vi "Multiple spectra.vi"() -> (0 "error out":errorcluster)   [LabVIEW 2021, in "Ceyear.lvlib"]
uses:
  <instrlib>/Ceyear/Ceyear.lvlib
  <instrlib>/Ceyear/Public/Configure/Configure lbd (Start Stop).vi
  <vilib>/Utility/file.llb/Write To Spreadsheet File (string).vi
  <instrlib>/Keithley 24XX/Keithley 24XX.lvlib
panel:
  in  "reverce":bool
  out "appended array":string[][](array[string])
  in  "Array smsr":dbl[](array[numeric])
  in  "Array 2nd peak wl":dbl[](array[numeric])
  in  "Array 1st peak wl":dbl[](array[numeric])
  in  "Limit [V]":dbl=4.0 format="%#.4f"
  out "keithly2400 connection":bool
  out "VCSEL error":errorcluster
  in  "VCSEL Serial Configuration":T1={"Baud Rate"=9600, "Parity"=0, "Data Bits"=8, "Stop Bits"=10, "Flow Control"=0} {"Flow Control" items=["None", "XON/XOFF", "RTS/CTS", "XON/XOFF & RTS/CTS", "DTR/DSR", "XON/XOFF & DTR/DSR"]; "Stop Bits" items=["1.0"=10, "1.5"=15, "2.0"=20]; "Data Bits" items=["7"=7, "8"=8]; "Parity" items=["None", "Odd", "Even", "Mark", "Space"]; "Baud Rate" items=["300"=300, "600"=600, "1200"=1200, "2400"=2400, "4800"=4800, "9600"=9600, "19200"=19200]}
  in  "VCSEL VISA resource name":refnum<visa-resource-name>="GPIB0::26::INSTR"
  in  "Exit":bool
  in  "osa_time_array":dbl[](array[numeric])=[950.0, 1350.0, 4400.0, 7500.0, 65600.0]
  out "Estimated time, min":dbl
  out "scale":u16(ring)=1 items=["LIN", "LOG"]
  out "Graphs array":cluster{"ArrayX":dbl[], "ArrayY":dbl[]}[](array[cluster]) {"ArrayY" format="%.2f"; "ArrayX" format="%.2f"}
  in  "current graph":u16(ring) items=["1", "2", "3", "4", "5"]
  out "ArrayY":dbl[](array[numeric])
  out "ArrayX":dbl[](array[numeric])
  out "VISA out":refnum<visa-resource-name>
  in  "start array meas":bool
  out "Progress":u8(slide) scale=0.0..100.0
  in  "Delete [mA]":dbl=0.5 caption="delete [mA]" format="%#.6f"
  in  "Delete":bool
  in  "Append":bool
  in  "Change":bool
  in  "Add [mA]":dbl=0.5 caption="add [mA]" format="%#.6f"
  out "Current meas array":dbl[](array[numeric])
  out "Points LVI":i32=21 caption="Points"
  in  "Step [mA] LVI":dbl=0.2 caption="Step [mA]" format="%#.10f"
  in  "Start [mA] LVI":dbl=0.1 caption="Start [mA]" format="%#.6f"
  in  "Stop [mA] LVI":dbl=4.1 caption="Stop [mA]" format="%#.2f"
  in  "single":bool
  in  "dl resolution, nm":u16(ring)=2 items=["0.02", "0.05", "0.1", "0.2", "0.5", "1", "2"]
  in  "apply":bool
  in  "sampling point":i32=2001
  in  "average times":i32=1
  in  "trace Read/Measurement":u16(ring) items=["Trace A", "Trace B", "Trace C", "Trace D", "Trace E"]
  in  "sensivity":u16(ring) items=["NORMAL", "MID", "HIGH1", "HIGH2", "HIGH3"]
  in  "L max (nm)":dbl=900.0 format="%.2f"
  in  "L min (nm)":dbl=880.0 format="%.2f"
  in  "Selecting folder LIV":path=path "Select Folder" caption="Selecting folder"
  in  "save":bool
  in  "Filename peak wl":string="OS_peak_wl"
  in  "Filename smsr":string="OS_smsr"
  in  "Filename all spectra":string="OS_all_spectra"
  in  "save peak wl":bool=TRUE
  in  "save smsr":bool=TRUE
  in  "save all spectra data":bool=TRUE
  out "SMSR":cluster{"Current meas array":dbl[], dbl[]}(graph)
  out "peak wl":cluster{"Current meas array":dbl[], dbl[]}[](graph)
  out "All spectras":cluster{"ArrayX":dbl[], "ArrayY":dbl[]}[](graph)
  # "OSA trace parameters"
  # "optical input 600--1700 nm"
  # "101-50001 points"
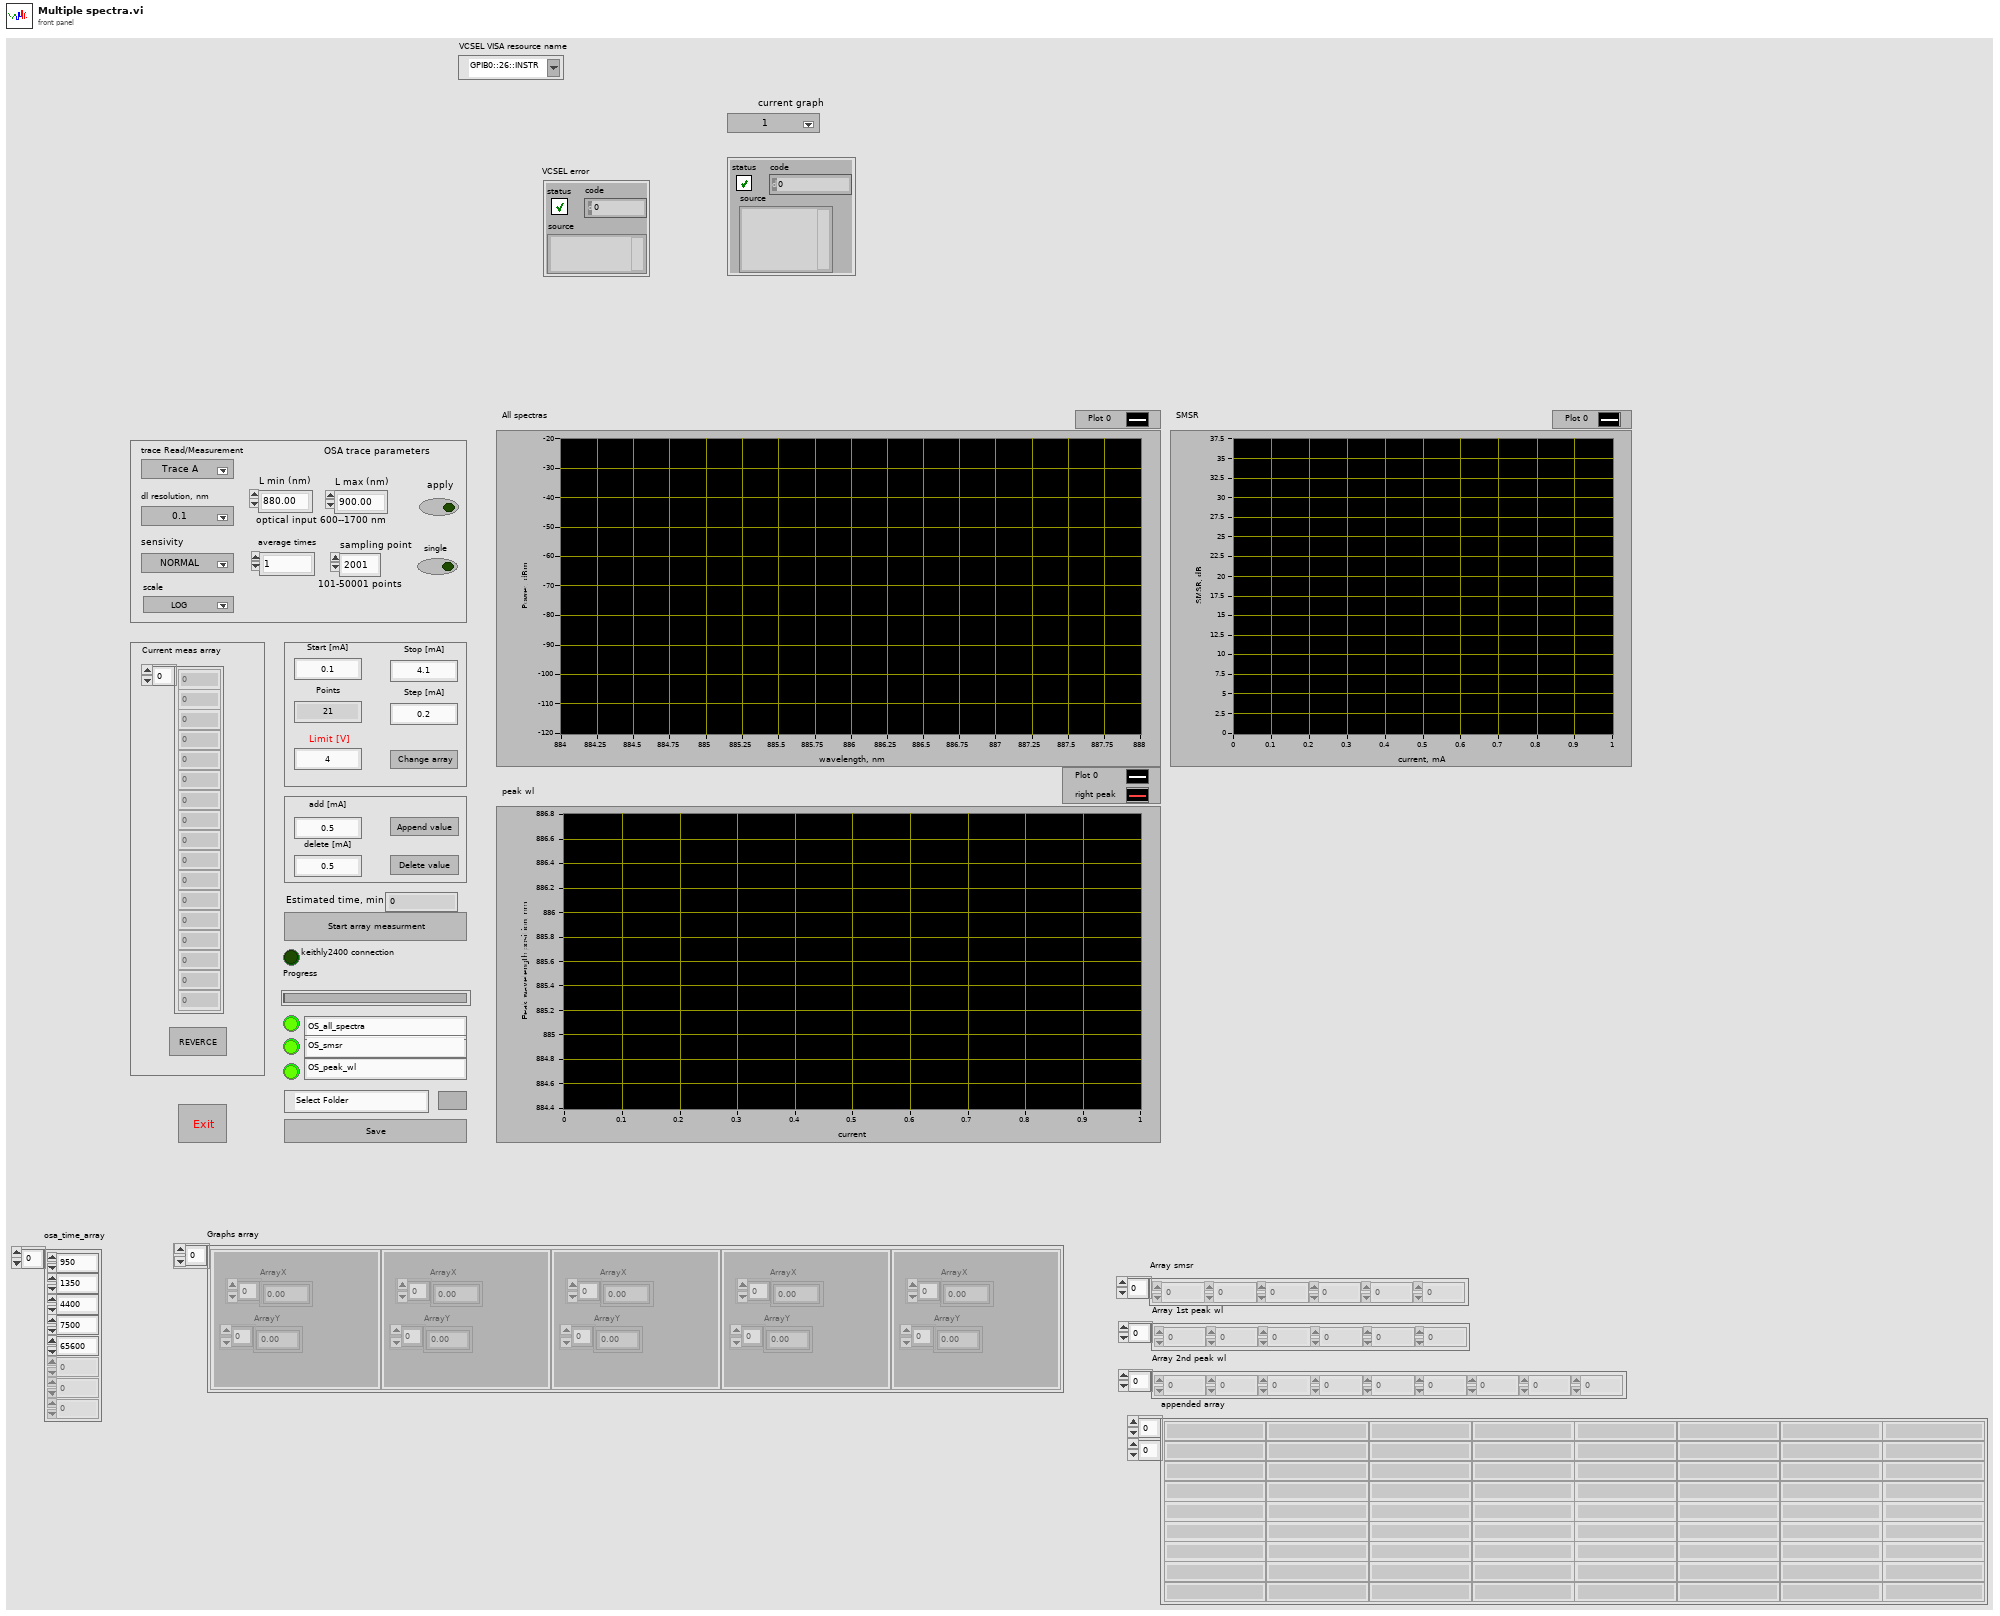
[diagram p1: front panel]
types:
  T1 = cluster{"Baud Rate":u32, "Parity":u16, "Data Bits":u16, "Stop Bits":u16, "Flow Control":u16}
  T2 = enum16{"Left Button", "Center Button", "Right Button", "Window Close"}
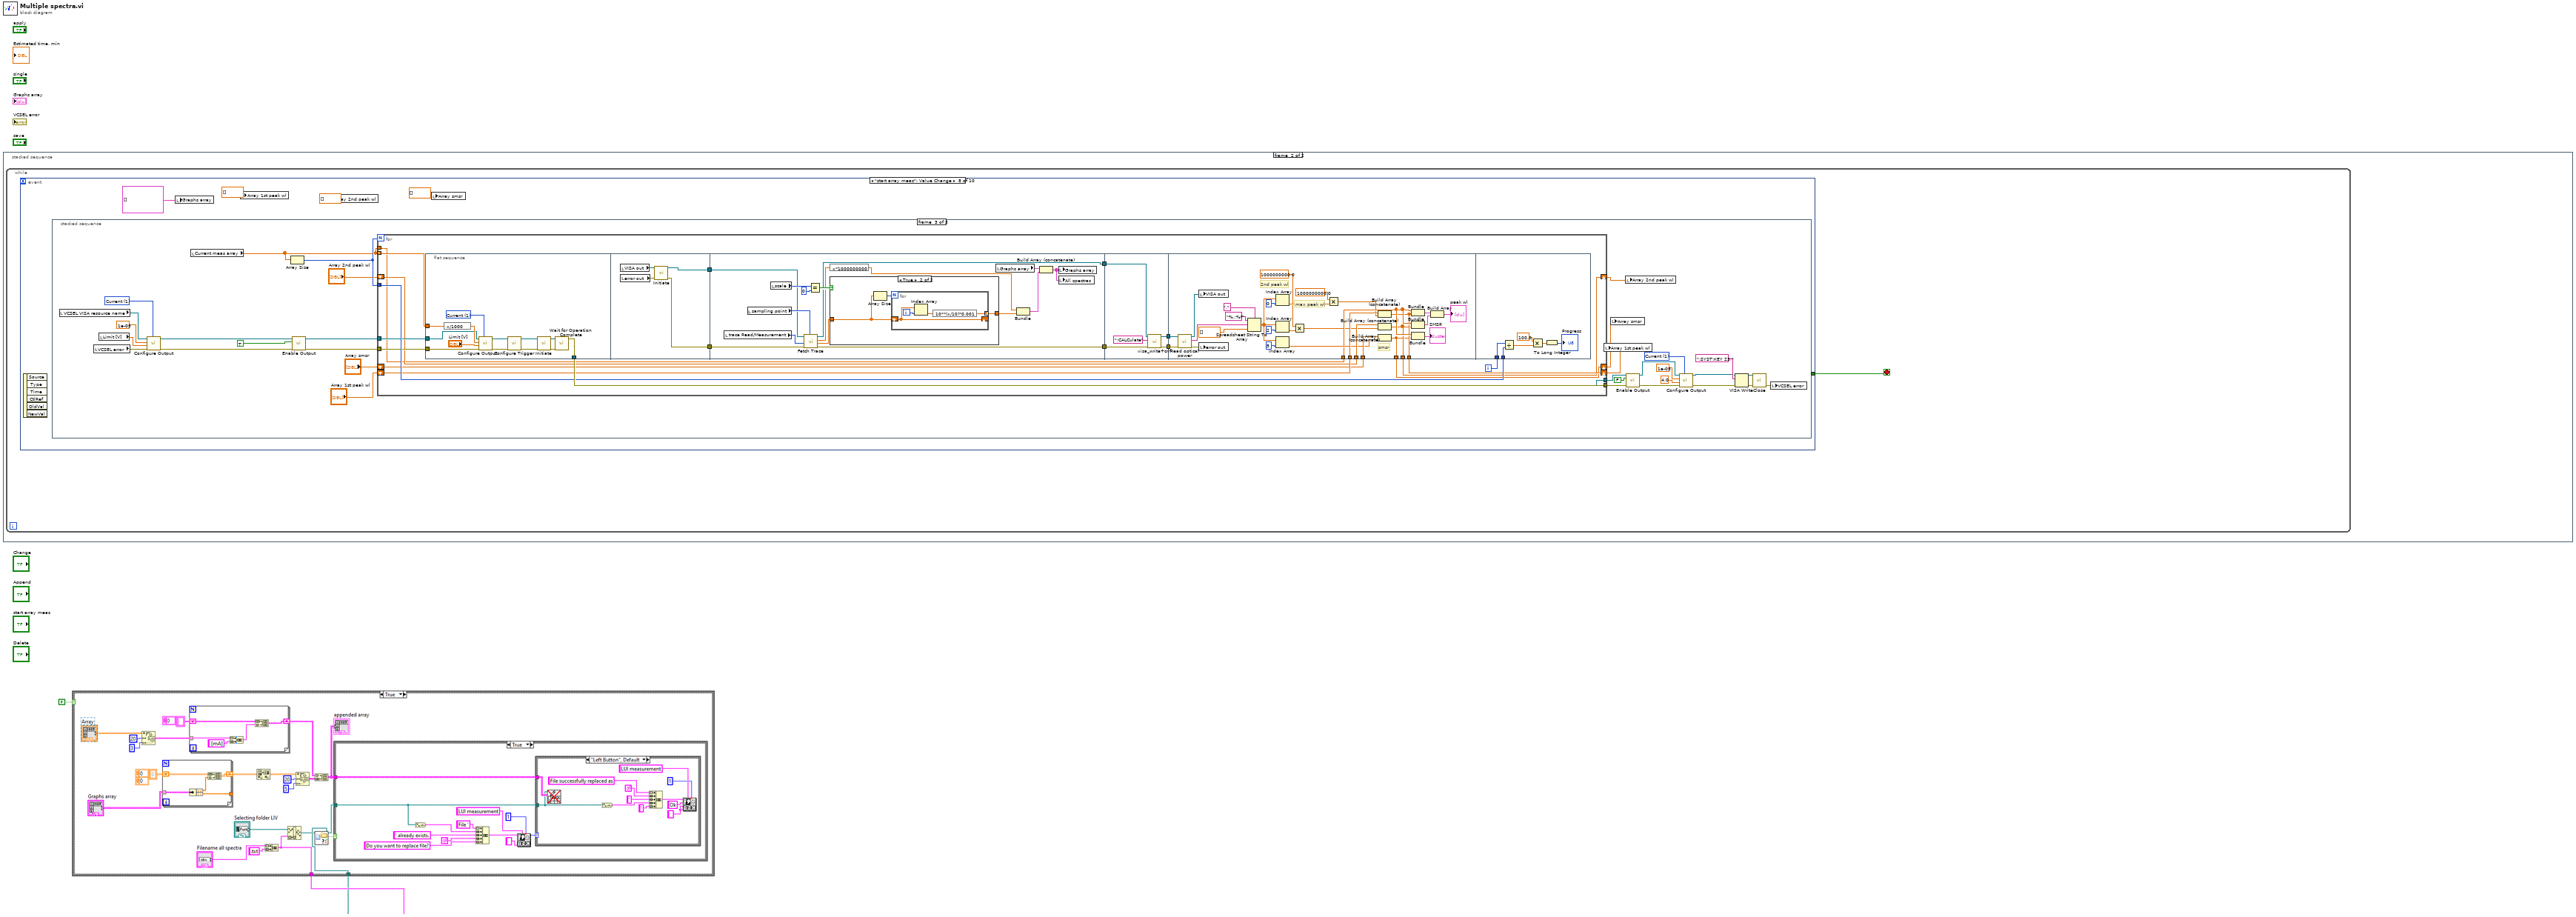
[diagram p0: block diagram]
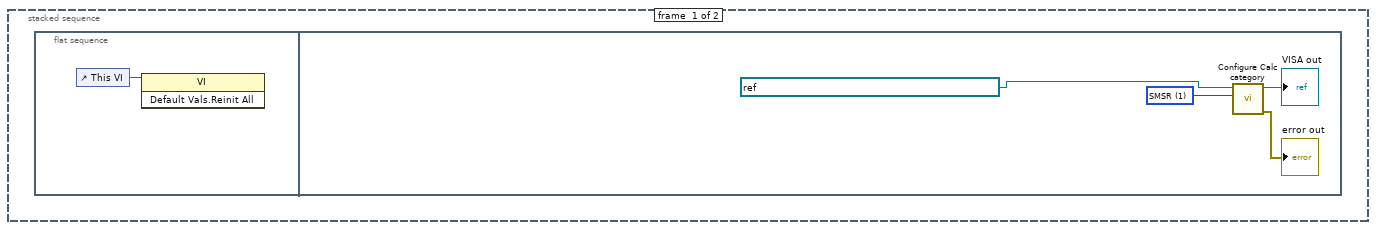
[diagram p2: hidden frame]
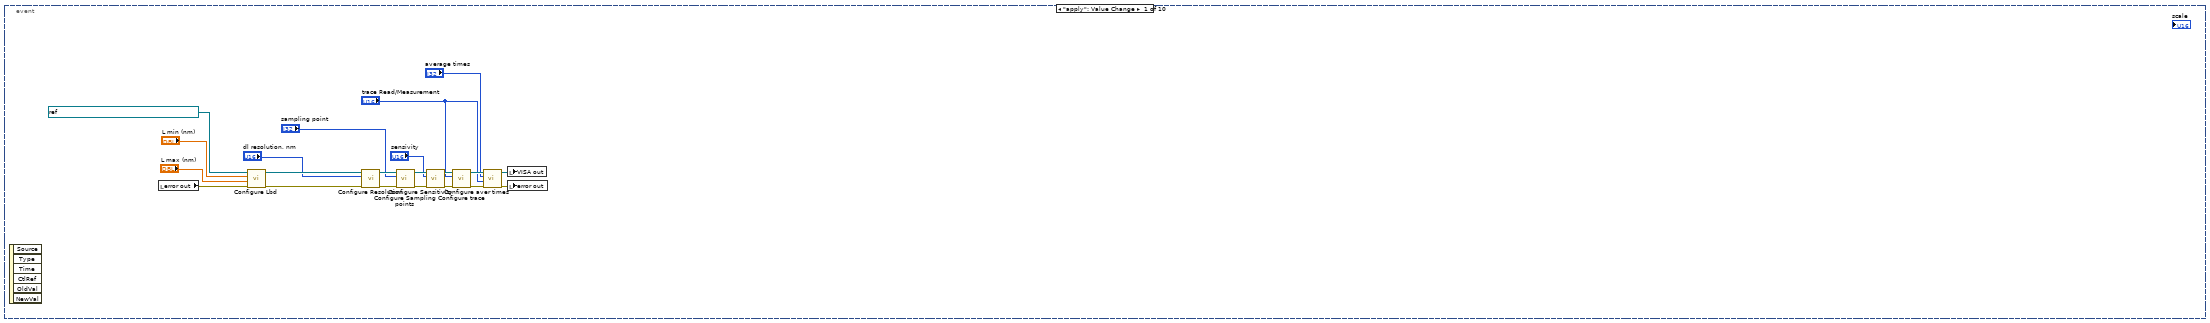
[diagram p3: hidden frame]
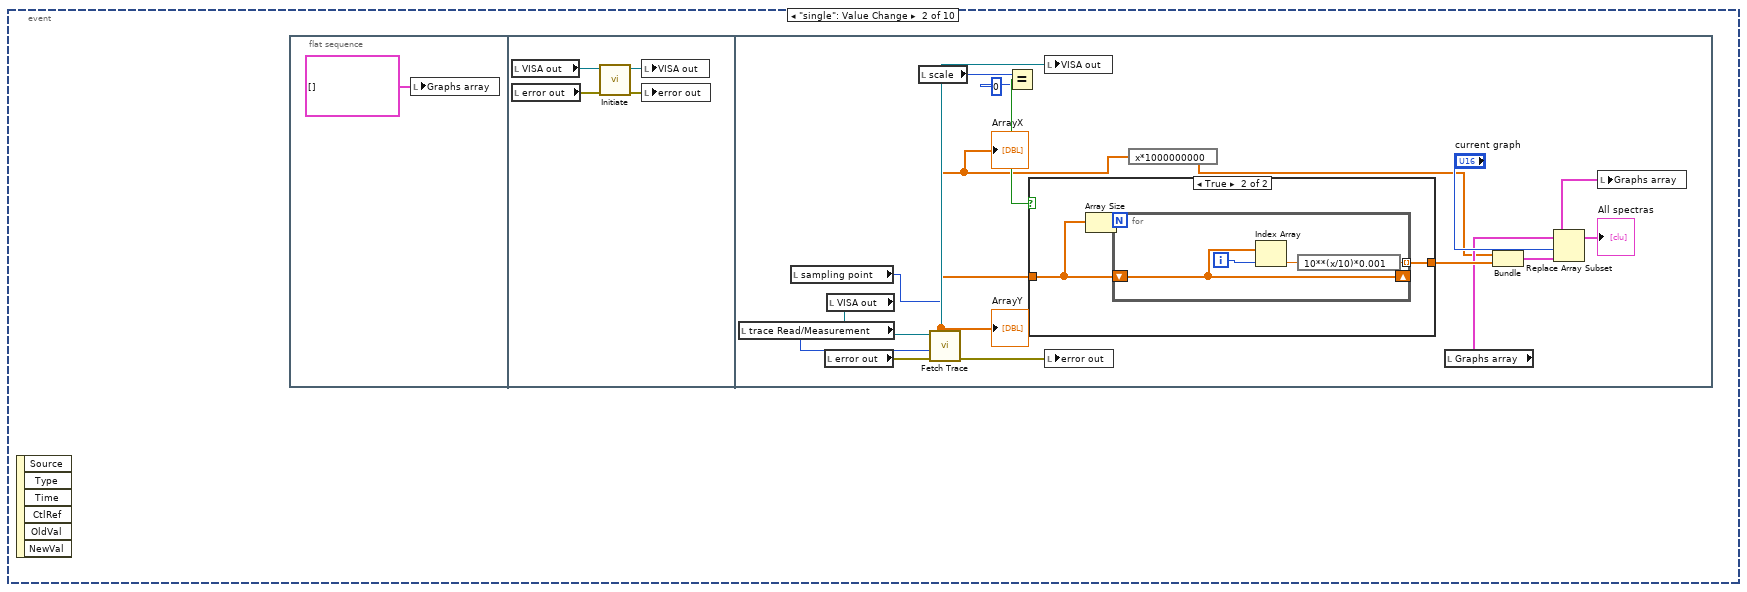
[diagram p4: hidden frame]
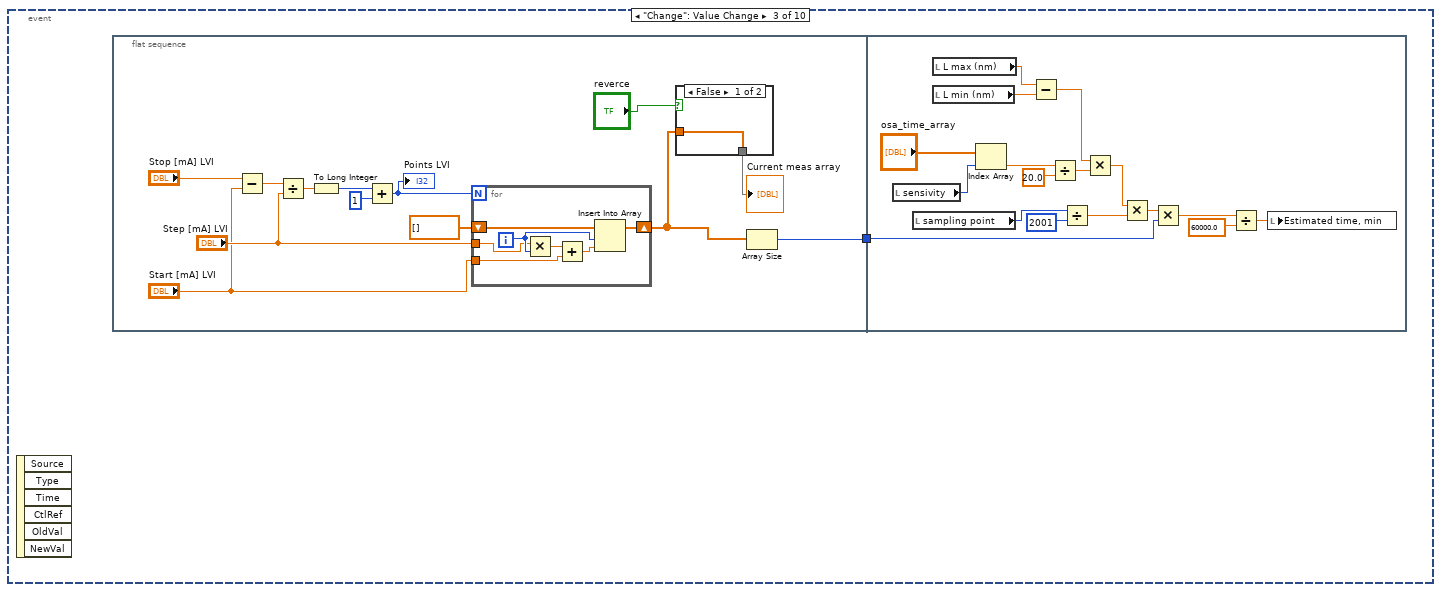
[diagram p6: hidden frame]
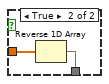
[diagram p7: hidden frame]
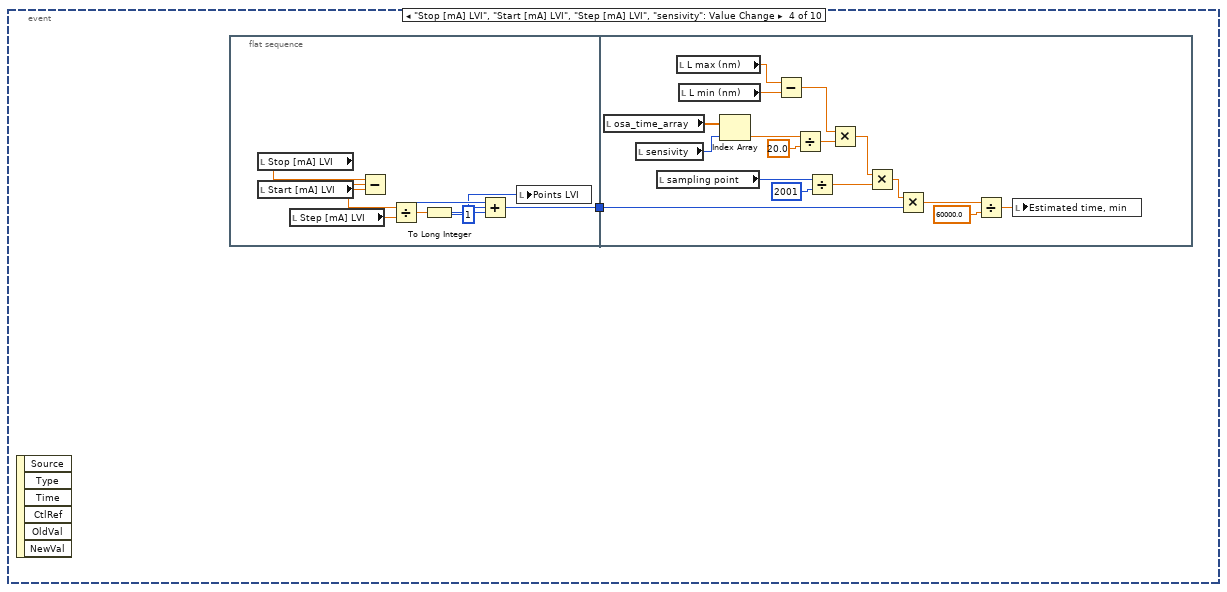
[diagram p8: hidden frame]
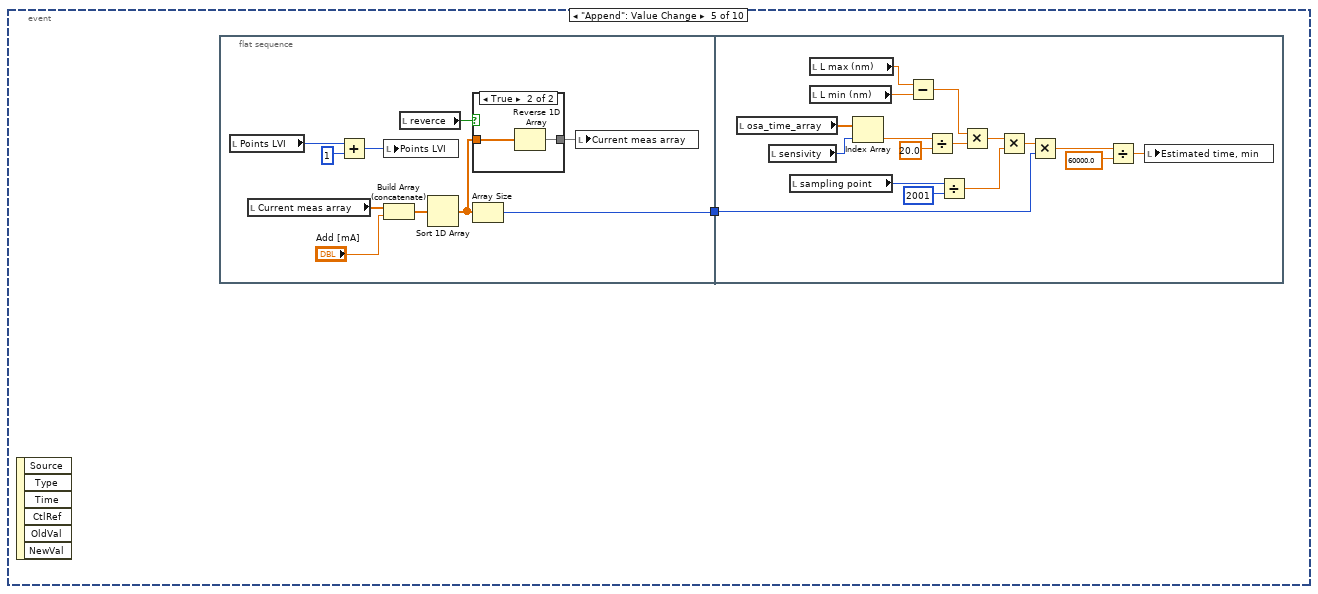
[diagram p9: hidden frame]
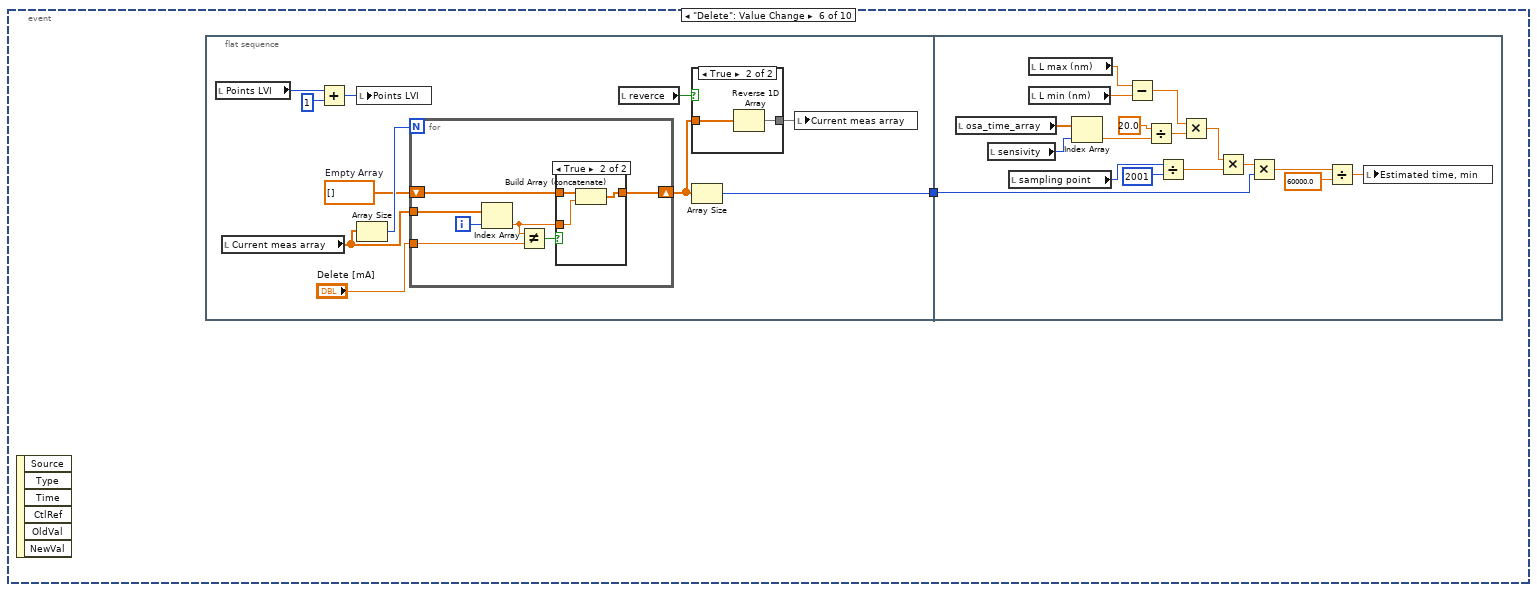
[diagram p11: hidden frame]
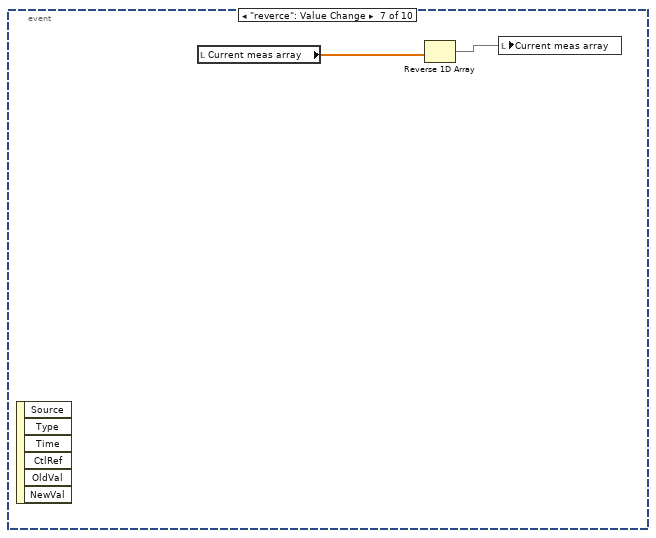
[diagram p14: hidden frame]
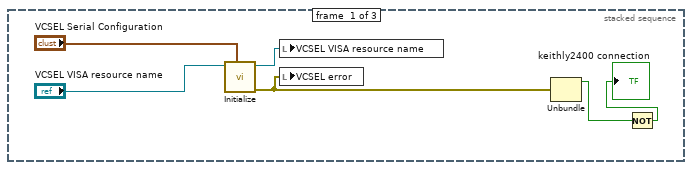
[diagram p15: hidden frame]
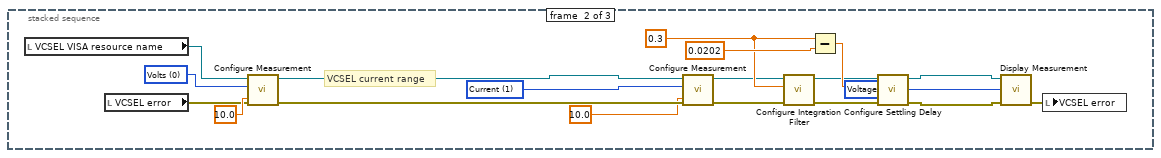
[diagram p16: hidden frame]
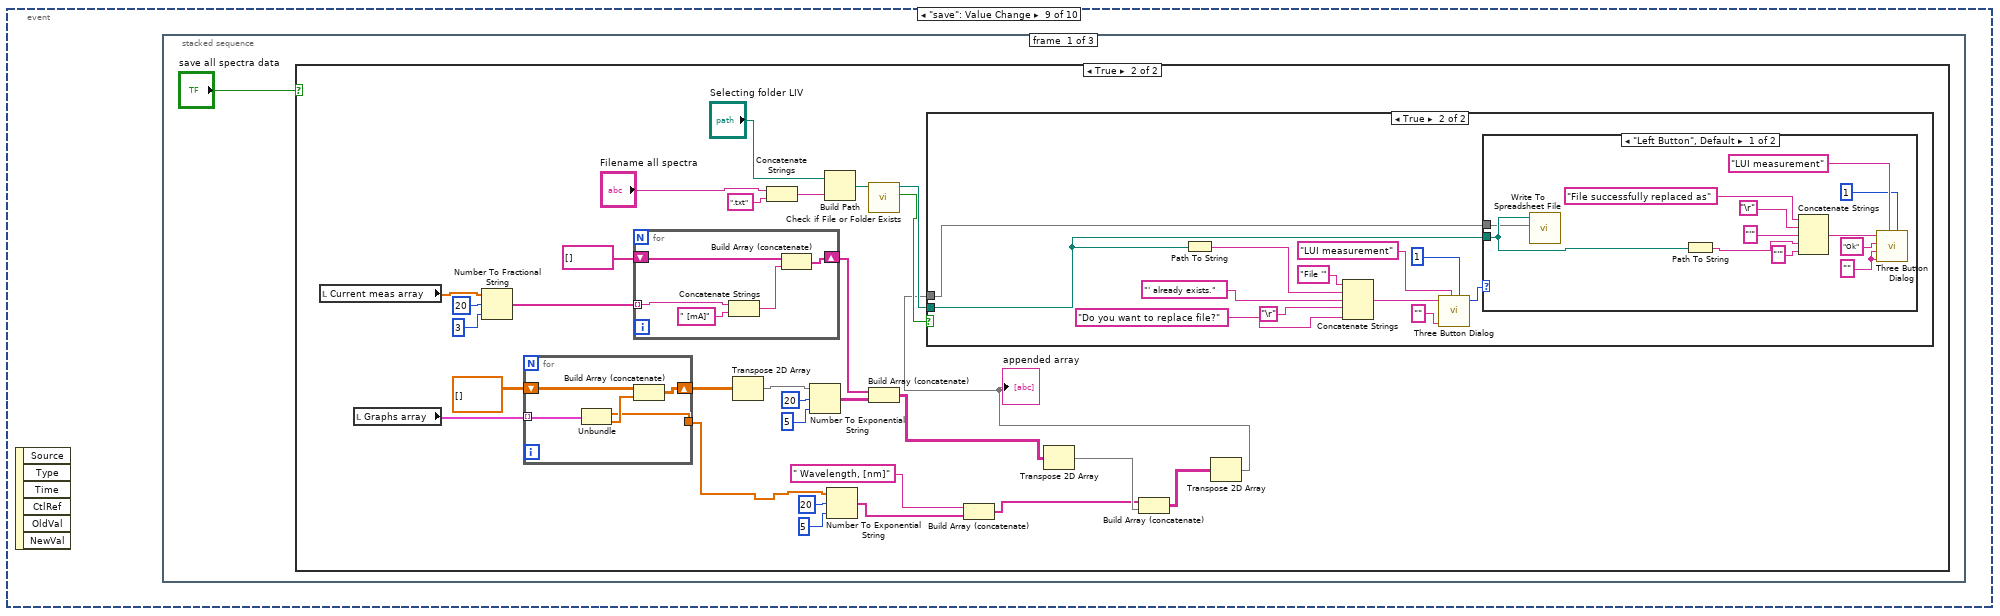
[diagram p18: hidden frame]
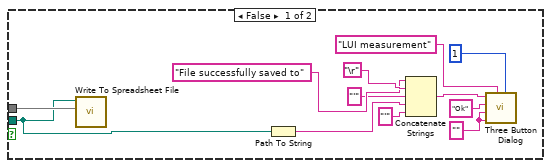
[diagram p20: hidden frame]
diagram:
  n1 = stacked-sequence {
    frame #0 {
      n2 = flat-sequence {
        frame #0 {
          n3 = control-ref of="This VI"() -> (w1:refnum<vi>)
          n4 = invoke class="VI" method="Default Vals.Reinit All"(reference=w1) -> ()  [unwired: 2 in, 3 out]
        }
        frame #1 {
          w5 = u16 1 items=["Power", "SMSR"] ("Category")
          n5 = call <instrlib>:"Configure Calc category.vi"("Category"=w5, "VISA resource name"=refnum<visa-resource-name> "TCPIP0::192.168.5.110::10001::SOCKET") -> ("error out"=→"error out":errorcluster, "VISA resource name out"=→"VISA out":refnum<visa-resource-name>)  [unwired: 7 in, 1 out]
        }
      }
    }
    frame #1 {
      n6 = while {
        stop <- w6 stop-if-true
        n7 = event shown="[7] \"start array meas\": Value Change" {
          selector: _ -> [_ _ _ _ _ _ _ _ _ _]
          dyn-events: _ -> [_ _ _ _ _ _ _ _ _ _]
          timeout: _ -> [_ _ _ _ _ _ _ _ _ _]
          tunnel: [_ _ _ _ _ _ _ _ _ w564] -> w6
          event "apply": Value Change {
            n8 = event-data() -> ()  [unwired: 1 in, 6 out]
            n9 = local read "error out"() -> (w15:errorcluster)
            n10 = call-poly <instrlib>:"Configure Lbd.vi"("error in (no error)"=w15, "Stop Frequency (nm)"="L max (nm)", "Start Frequency (nm)"="L min (nm)", "VISA resource name"=refnum<visa-resource-name> "TCPIP0::192.168.5.110::10001::SOCKET") -> ("error out"=w27:errorcluster, "VISA resource name out"=w22:refnum<visa-resource-name>)  [unwired: 6 in]
            n11 = call <instrlib>:"Configure Resolution.vi"("error in (no error)"=w27, "Resolution (nm)"="dl resolution, nm", "VISA resource name"=w22) -> ("error out"=w26:errorcluster, "VISA resource name out"=w23:refnum<visa-resource-name>)  [unwired: 7 in]
            n12 = call <instrlib>:"Configure Sampling points.vi"("error in (no error)"=w26, "Sampling points"="sampling point", "VISA resource name"=w23) -> ("error out"=w25:errorcluster, "VISA resource name out"=w24:refnum<visa-resource-name>)  [unwired: 7 in]
            n13 = call <instrlib>:"Configure Sensitivity.vi"("error in (no error)"=w25, "Sensse mode"="sensivity", "VISA resource name"=w24) -> ("error out"=w17:errorcluster, "VISA resource name out"=w16:refnum<visa-resource-name>)  [unwired: 7 in]
            n14 = call <instrlib>:"Configure trace.vi"("error in (no error)"=w17, "Trace"="trace Read/Measurement", "VISA resource name"=w16) -> ("error out"=w19:errorcluster, "VISA resource name out"=w18:refnum<visa-resource-name>)  [unwired: 7 in]
            n15 = call <instrlib>:"Configure aver times.vi"("error in (no error)"=w19, "Trace"="trace Read/Measurement", "Averaging times"="average times", "VISA resource name"=w18) -> ("error out"=w21:errorcluster, "VISA resource name out"=w20:refnum<visa-resource-name>)  [unwired: 6 in]
            n16 = local write "VISA out"(w20) -> ()
            n17 = local write "error out"(w21) -> ()
          }
          event "single": Value Change {
            n18 = event-data() -> ()  [unwired: 1 in, 6 out]
            n19 = flat-sequence {
              frame #0 {
                n20 = local write "Graphs array"(cluster{"ArrayX":dbl[], "ArrayY":dbl[]}[] [] ("Graphs array")) -> ()
              }
              frame #1 {
                n21 = local read "VISA out"() -> (w32:refnum<visa-resource-name>)
                n22 = local read "error out"() -> (w31:errorcluster)
                n23 = call <instrlib>:"Initiate.vi"("error in (no error)"=w31, "VISA resource name"=w32) -> ("error out"=w29:errorcluster, "VISA resource name out"=w30:refnum<visa-resource-name>)  [unwired: 8 in]
                n24 = local write "VISA out"(w30) -> ()
                n25 = local write "error out"(w29) -> ()
              }
              frame #2 {
                n26 = local read "trace Read/Measurement"() -> (w48:u16)
                n27 = local read "sampling point"() -> (w40:i32)
                n28 = local read "error out"() -> (w46:errorcluster)
                n29 = local read "VISA out"() -> (w47:refnum<visa-resource-name>)
                n30 = local read "scale"() -> (w42:u16)
                n31 = call <instrlib>:"Fetch Trace.vi"("Points"=w40, "error in (no error)"=w46, "Trace"=w48, "VISA resource name"=w47) -> ("error out"=w44:errorcluster, "Y array"=w43:dbl[], "X array"=w35:dbl[], "VISA resource name out"=w45:refnum<visa-resource-name>)  [unwired: 4 in]
                "ArrayX" <- w35
                "ArrayY" <- w43
                n32 = Equal?(x=w42, y=0) -> (x = y?=w41:bool)
                n33 = case shown="True" w41 {
                  tunnel: w43 -> [w50 w52]
                  tunnel: [w50 w51] -> w38
                  frame False {
                  }
                  frame True {
                    n34 = Array Size(array=w52) -> (size(s)=w53:i32)
                    n35 = for {
                      N: w53 -> [_]
                      shift-right: [w56] -> _
                      shift-left: w52 -> [w56]
                      tunnel: [w54] -> w51 mode=indexing
                      i -> [w57]
                      n36 = Index Array(array=w56, index=w57) -> (element=w55:dbl)
                      n37 = expression code="10**(x/10)*0.001"(w55) -> (w54:dbl)
                    }
                  }
                }
                n38 = local write "VISA out"(w45) -> ()
                n39 = local write "error out"(w44) -> ()
                n40 = expression code="x*1000000000"(w35) -> (w34:dbl[])
                n41 = local read "Graphs array"() -> (w37:cluster{"ArrayX":dbl[], "ArrayY":dbl[]}[])
                n42 = Bundle("X array"=w34, "Y array"=w38) -> (w36:cluster{"X array":dbl[], "Y array":dbl[]})  [unwired: 1 in]
                n43 = Replace Array Subset(array=w37, new element=w36, index="current graph") -> (w49:cluster{"ArrayX":dbl[], "ArrayY":dbl[]}[])
                "All spectras" <- w49
                n44 = local write "Graphs array"(w49) -> ()
              }
            }
          }
          event "Change": Value Change {
            n45 = event-data() -> ()  [unwired: 1 in, 6 out]
            n46 = flat-sequence {
              tunnel: [w67] -> w58
              tunnel: w58 -> [w98]
              frame #0 {
                n47 = Subtract(x="Stop [mA] LVI", y="Start [mA] LVI") -> (x-y=w70:dbl)
                n48 = Divide(x=w70, y="Step [mA] LVI") -> (x/y=w68:dbl)
                n49 = To Long Integer(number=w68) -> (32bit integer=w63:i32)
                n50 = Add(x=w63, y=1) -> (x+y=w64:i32)
                "Points LVI" <- w64
                n51 = for {
                  N: w64 -> [_]
                  shift-right: [w78] -> w61
                  shift-left: dbl[] [] ("Current meas array") -> [w81]
                  tunnel: "Step [mA] LVI" -> [w79]
                  tunnel: "Start [mA] LVI" -> [w76]
                  i -> [w80]
                  n52 = Multiply(x=w79, y=w80) -> (x*y=w77:dbl)
                  n53 = Add(x=w77, y=w76) -> (x+y=w75:dbl)
                  n54 = Insert Into Array(array=w81, index=w80, new element=w75) -> (w78:dbl[])
                }
                n55 = case shown="False" "reverce" {
                  tunnel: w61 -> [w72 w74]
                  tunnel: [w72 w73] -> w60
                  frame False {
                  }
                  frame True {
                    n56 = Reverse 1D Array(array=w74) -> (reversed array=w73:dbl[])
                  }
                }
                "Current meas array" <- w60
                n57 = Array Size(array=w61) -> (size(s)=w67:i32)
              }
              frame #1 {
                n58 = local read "sensivity"() -> (w90:u16)
                n59 = local read "sampling point"() -> (w82:i32)
                n60 = local read "L max (nm)"() -> (w92:dbl)
                n61 = local read "L min (nm)"() -> (w93:dbl)
                n62 = Index Array(array="osa_time_array", index=w90) -> (element=w84:dbl)
                n63 = Subtract(x=w92, y=w93) -> (x-y=w94:dbl)
                n64 = Divide(x=w84, y=20.0 ("x")) -> (x/y=w95:dbl)
                n65 = Divide(x=w82, y=2001) -> (x/y=w96:dbl)
                n66 = Multiply(x=w94, y=w95) -> (x*y=w97:dbl)
                n67 = Multiply(x=w97, y=w96) -> (x*y=w89:dbl)
                n68 = Multiply(x=w89, y=w98) -> (x*y=w87:dbl)
                n69 = Divide(x=w87, y=60000.0) -> (x/y=w86:dbl)
                n70 = local write "Estimated time, min"(w86) -> ()
              }
            }
          }
          event "Stop [mA] LVI", "Start [mA] LVI", "Step [mA] LVI", "sensivity": Value Change {
            n71 = event-data() -> ()  [unwired: 1 in, 6 out]
            n72 = flat-sequence {
              tunnel: [w100] -> w99
              tunnel: w99 -> [w124]
              frame #0 {
                n73 = local read "Stop [mA] LVI"() -> (w105:dbl)
                n74 = local read "Start [mA] LVI"() -> (w103:dbl)
                n75 = local read "Step [mA] LVI"() -> (w104:dbl)
                n76 = Subtract(x=w105, y=w103) -> (x-y=w107:dbl)
                n77 = Divide(x=w107, y=w104) -> (x/y=w106:dbl)
                n78 = To Long Integer(number=w106) -> (32bit integer=w101:i32)
                n79 = Add(x=w101, y=1) -> (x+y=w100:i32)
                n80 = local write "Points LVI"(w100) -> ()
              }
              frame #1 {
                n81 = local read "osa_time_array"() -> (w112:dbl[])
                n82 = local read "sensivity"() -> (w117:u16)
                n83 = local read "sampling point"() -> (w108:i32)
                n84 = local read "L max (nm)"() -> (w118:dbl)
                n85 = local read "L min (nm)"() -> (w119:dbl)
                n86 = Index Array(array=w112, index=w117) -> (element=w110:dbl)
                n87 = Subtract(x=w118, y=w119) -> (x-y=w120:dbl)
                n88 = Divide(x=w110, y=20.0 ("x")) -> (x/y=w121:dbl)
                n89 = Divide(x=w108, y=2001) -> (x/y=w122:dbl)
                n90 = Multiply(x=w120, y=w121) -> (x*y=w123:dbl)
                n91 = Multiply(x=w123, y=w122) -> (x*y=w116:dbl)
                n92 = Multiply(x=w116, y=w124) -> (x*y=w114:dbl)
                n93 = Divide(x=w114, y=60000.0) -> (x/y=w113:dbl)
                n94 = local write "Estimated time, min"(w113) -> ()
              }
            }
          }
          event "Append": Value Change {
            n95 = event-data() -> ()  [unwired: 1 in, 6 out]
            n96 = flat-sequence {
              tunnel: [w133] -> w125
              tunnel: w125 -> [w155]
              frame #0 {
                n97 = local read "Points LVI"() -> (w132:i32)
                n98 = local read "Current meas array"() -> (w134:dbl[])
                n99 = Add(x=w132, y=1) -> (x+y=w130:i32)
                n100 = local write "Points LVI"(w130) -> ()
                n101 = Build Array (concatenate)(w134, "Add [mA]") -> (w129:dbl[])
                n102 = local read "reverce"() -> (w126:bool)
                n103 = Sort 1D Array(array=w129) -> (sorted array=w128:dbl[])
                n104 = case shown="True" w126 {
                  tunnel: w128 -> [w136 w138]
                  tunnel: [w136 w137] -> w127
                  frame False {
                  }
                  frame True {
                    n105 = Reverse 1D Array(array=w138) -> (reversed array=w137:dbl[])
                  }
                }
                n106 = Array Size(array=w128) -> (size(s)=w133:i32)
                n107 = local write "Current meas array"(w127) -> ()
              }
              frame #1 {
                n108 = local read "osa_time_array"() -> (w147:dbl[])
                n109 = local read "sensivity"() -> (w146:u16)
                n110 = local read "sampling point"() -> (w139:i32)
                n111 = local read "L max (nm)"() -> (w144:dbl)
                n112 = local read "L min (nm)"() -> (w143:dbl)
                n113 = Index Array(array=w147, index=w146) -> (element=w141:dbl)
                n114 = Subtract(x=w144, y=w143) -> (x-y=w151:dbl)
                n115 = Divide(x=w141, y=20.0 ("x")) -> (x/y=w152:dbl)
                n116 = Divide(x=w139, y=2001) -> (x/y=w153:dbl)
                n117 = Multiply(x=w151, y=w152) -> (x*y=w154:dbl)
                n118 = Multiply(x=w154, y=w153) -> (x*y=w145:dbl)
                n119 = Multiply(x=w145, y=w155) -> (x*y=w149:dbl)
                n120 = Divide(x=w149, y=60000.0) -> (x/y=w148:dbl)
                n121 = local write "Estimated time, min"(w148) -> ()
              }
            }
          }
          event "Delete": Value Change {
            n122 = event-data() -> ()  [unwired: 1 in, 6 out]
            n123 = flat-sequence {
              tunnel: [w163] -> w156
              tunnel: w156 -> [w187]
              frame #0 {
                w165 = dbl[] []  # Empty Array
                n124 = local read "Points LVI"() -> (w161:i32)
                n125 = local read "Current meas array"() -> (w166:dbl[])
                n126 = Add(x=w161, y=1) -> (x+y=w160:i32)
                n127 = local write "Points LVI"(w160) -> ()
                n128 = Array Size(array=w166) -> (size(s)=w167:i32)
                n129 = for {
                  N: w167 -> [_]
                  shift-right: [w172] -> w159
                  shift-left: w165 -> [w173]
                  tunnel: w166 -> [w177]
                  tunnel: "Delete [mA]" -> [w175]
                  i -> [w176]
                  n130 = Index Array(array=w177, index=w176) -> (element=w171:dbl)
                  n131 = Not Equal?(x=w171, y=w175) -> (x != y?=w174:bool)
                  n132 = case shown="True" w174 {
                    tunnel: w173 -> [w178 w181]
                    tunnel: [w178 w180] -> w172
                    tunnel: w171 -> [_ w179]
                    frame False {
                    }
                    frame True {
                      n133 = Build Array (concatenate)(w181, w179) -> (w180:dbl[])
                    }
                  }
                }
                n134 = local read "reverce"() -> (w157:bool)
                n135 = case shown="True" w157 {
                  tunnel: w159 -> [w168 w170]
                  tunnel: [w168 w169] -> w158
                  frame False {
                  }
                  frame True {
                    n136 = Reverse 1D Array(array=w170) -> (reversed array=w169:dbl[])
                  }
                }
                n137 = Array Size(array=w159) -> (size(s)=w163:i32)
                n138 = local write "Current meas array"(w158) -> ()
              }
              frame #1 {
                n139 = local read "osa_time_array"() -> (w189:dbl[])
                n140 = local read "sensivity"() -> (w188:u16)
                n141 = local read "sampling point"() -> (w182:i32)
                n142 = local read "L max (nm)"() -> (w191:dbl)
                n143 = local read "L min (nm)"() -> (w190:dbl)
                n144 = Index Array(array=w189, index=w188) -> (element=w184:dbl)
                n145 = Subtract(x=w191, y=w190) -> (x-y=w195:dbl)
                n146 = Divide(x=20.0, y=w184) -> (x/y=w196:dbl)
                n147 = Divide(x=w182, y=2001) -> (x/y=w197:dbl)
                n148 = Multiply(x=w195, y=w196) -> (x*y=w198:dbl)
                n149 = Multiply(x=w198, y=w197) -> (x*y=w192:dbl)
                n150 = Multiply(x=w192, y=w187) -> (x*y=w193:dbl)
                n151 = Divide(x=w193, y=60000.0) -> (x/y=w186:dbl)
                n152 = local write "Estimated time, min"(w186) -> ()
              }
            }
          }
          event "reverce": Value Change {
            n153 = event-data() -> ()  [unwired: 1 in, 6 out]
            n154 = local read "Current meas array"() -> (w200:dbl[])
            n155 = Reverse 1D Array(array=w200) -> (reversed array=w199:dbl[])
            n156 = local write "Current meas array"(w199) -> ()
          }
          event "start array meas": Value Change {
            n157 = event-data() -> ()  [unwired: 1 in, 6 out]
            n158 = stacked-sequence {
              frame #0 {
                n159 = call <instrlib>:"Initialize.vi"("Serial Configuration"="VCSEL Serial Configuration", "VISA resource name"="VCSEL VISA resource name") -> ("error out"=w207:errorcluster, "VISA resource name out"=w208:refnum<visa-resource-name>)  [unwired: 3 in, 5 out]
                n160 = local write "VCSEL VISA resource name"(w208) -> ()
                n161 = local write "VCSEL error"(w207) -> ()
                n162 = Unbundle(w207) -> ("status"=w206:bool)  [unwired: 2 out]
                n163 = Not(x=w206) -> (.not. x?=→"keithly2400 connection":bool)
              }
              frame #1 {
                w223 = 0.3
                w215 = u16 0 items=["Voltage", "Current", "Resistance"] ("Displayed Measurement (0: Voltage)")
                w214 = u16 0 items=["Volts", "Current", "Resistance"] ("Function (0: Volts)")
                w225 = u16 1 items=["Voltage", "Current"] ("Source Mode  (0: Voltage)")
                # "VCSEL current range"
                n164 = local read "VCSEL VISA resource name"() -> (w221:refnum<visa-resource-name>)
                n165 = local read "VCSEL error"() -> (w219:errorcluster)
                n166 = call <instrlib>:"Configure Measurement.vi"("Manual Range (1.0)"=10.0, "error in (no error)"=w219, "Function (0: Volts)"=w214, "VISA resource name"=w221) -> ("error out"=w228:errorcluster, "VISA resource name out"=w229:refnum<visa-resource-name>)  [unwired: 6 in]
                n167 = call <instrlib>:"Configure Measurement.vi"("Manual Range (1.0)"=10.0, "error in (no error)"=w228, "Function (0: Volts)"=w225, "VISA resource name"=w229) -> ("error out"=w212:errorcluster, "VISA resource name out"=w213:refnum<visa-resource-name>)  [unwired: 6 in]
                n168 = call <instrlib>:"Configure Integration Filter.vi"("error in (no error)"=w212, "Measurement Speed (1 PLC)"=w223, "VISA resource name"=w213) -> ("error out"=w216:errorcluster, "VISA resource name out"=w217:refnum<visa-resource-name>)  [unwired: 7 in]
                n169 = Subtract(x=w223, y=0.0202) -> (x-y=w222:dbl)
                n170 = call <instrlib>:"Configure Settling Delay.vi"("error in (no error)"=w216, "Manual Settling Delay (0 sec)"=w222, "VISA resource name"=w217) -> ("error out"=w226:errorcluster, "VISA resource name out"=w227:refnum<visa-resource-name>)  [unwired: 7 in]
                n171 = call <instrlib>:"Display Measurement.vi"("error in (no error)"=w226, "Displayed Measurement (0: Voltage)"=w215, "VISA resource name"=w227) -> ("error out"=w211:errorcluster)  [unwired: 7 in, 1 out]
                n172 = local write "VCSEL error"(w211) -> ()
              }
              frame #2 {
                w239 = u16 1 items=["Voltage", "Current"] ("Source Mode  (0: Voltage)")
                w257 = u16 1 items=["Voltage", "Current"] ("Source Mode  (0: Voltage)")
                n173 = local read "VCSEL VISA resource name"() -> (w247:refnum<visa-resource-name>)
                n174 = local read "VCSEL error"() -> (w246:errorcluster)
                n175 = local read "Limit [V]"() -> (w245:dbl)
                n176 = call <instrlib>:"Configure Output.vi"("Source Mode  (0: Voltage)"=w239, "error in (no error)"=w246, "Compliance  Level (0.1)"=w245, "Output Level (0)"=1e-05, "VISA resource name"=w247) -> ("error out"=w249:errorcluster, "VISA resource name out"=w248:refnum<visa-resource-name>)  [unwired: 5 in]
                n177 = local read "Current meas array"() -> (w242:dbl[])
                n178 = Array Size(array=w242) -> (size(s)=w258:i32)
                n179 = call <instrlib>:"Enable Output.vi"("error in (no error)"=w249, "Enable Output (T: Enable)"=TRUE, "VISA resource name"=w248) -> ("error out"=w250:errorcluster, "VISA resource name out"=w251:refnum<visa-resource-name>)  [unwired: 7 in]
                n180 = for {
                  N: w258 -> [_]
                  tunnel: [w275] -> w260
                  tunnel: [w280] -> w259
                  tunnel: w242 -> [w281] mode=indexing
                  tunnel: w258 -> [w278]
                  tunnel: w251 -> [w277]
                  tunnel: w250 -> [w276]
                  shift-right: [w270] -> w230
                  shift-left: "Array 1st peak wl" -> [w274]
                  shift-right: [w269] -> w232
                  shift-left: "Array 2nd peak wl" -> [w273]
                  shift-right: [w268] -> w231
                  shift-left: "Array smsr" -> [w272]
                  tunnel: w242 -> [w271]
                  i -> [w279]
                  n181 = flat-sequence {
                    tunnel: w281 -> [w293]
                    tunnel: [w283] -> w280
                    tunnel: w277 -> [w291]
                    tunnel: w276 -> [w290]
                    tunnel: [w282] -> w275
                    tunnel: [w297] -> w263
                    tunnel: [w296] -> w262
                    tunnel: [w303] -> w267
                    tunnel: [w302] -> w265
                    tunnel: w263 -> [w301]
                    tunnel: w262 -> [w300]
                    tunnel: w267 -> [w327]
                    tunnel: [w326] -> w266
                    tunnel: w265 -> [w324]
                    tunnel: [w325] -> w264
                    tunnel: w266 -> [w358]
                    tunnel: w274 -> [w346]
                    tunnel: w273 -> [w345]
                    tunnel: w272 -> [w344]
                    tunnel: w271 -> [w339]
                    tunnel: [w337] -> w270
                    tunnel: [w336] -> w269
                    tunnel: [w335] -> w268
                    tunnel: w264 -> [w357]
                    tunnel: w279 -> [w364]
                    tunnel: w278 -> [w363]
                    frame #0 {
                      w292 = u16 1 items=["Voltage", "Current"] ("Source Mode  (0: Voltage)")
                      n182 = expression code="x/1000"(w293) -> (w295:dbl)
                      n183 = call <instrlib>:"Configure Output.vi"("Source Mode  (0: Voltage)"=w292, "error in (no error)"=w290, "Compliance  Level (0.1)"="Limit [V]", "Output Level (0)"=w295, "VISA resource name"=w291) -> ("error out"=w284:errorcluster, "VISA resource name out"=w285:refnum<visa-resource-name>)  [unwired: 5 in]
                      n184 = call <instrlib>:"Configure Trigger.vi"("error in (no error)"=w284, "VISA resource name"=w285) -> ("error out"=w288:errorcluster, "VISA resource name out"=w286:refnum<visa-resource-name>)  [unwired: 8 in]
                      n185 = call <instrlib>:"Initiate.vi"("error in (no error)"=w288, "VISA resource name"=w286) -> ("error out"=w289:errorcluster, "VISA resource name out"=w287:refnum<visa-resource-name>)  [unwired: 8 in]
                      n186 = call <instrlib>:"Wait for Operation Complete.vi"("error in (no error)"=w289, "VISA resource name"=w287) -> ("error out"=w283:errorcluster, "VISA resource name out"=w282:refnum<visa-resource-name>)  [unwired: 8 in]
                    }
                    frame #1 {
                      n187 = local read "VISA out"() -> (w299:refnum<visa-resource-name>)
                      n188 = local read "error out"() -> (w298:errorcluster)
                      n189 = call <instrlib>:"Initiate.vi"("error in (no error)"=w298, "VISA resource name"=w299) -> ("error out"=w296:errorcluster, "VISA resource name out"=w297:refnum<visa-resource-name>)  [unwired: 8 in]
                    }
                    frame #2 {
                      n190 = local read "trace Read/Measurement"() -> (w315:u16)
                      n191 = local read "sampling point"() -> (w311:i32)
                      n192 = local read "scale"() -> (w313:u16)
                      n193 = call <instrlib>:"Fetch Trace.vi"("Points"=w311, "error in (no error)"=w300, "Trace"=w315, "VISA resource name"=w301) -> ("error out"=w302:errorcluster, "Y array"=w314:dbl[], "X array"=w309:dbl[], "VISA resource name out"=w303:refnum<visa-resource-name>)  [unwired: 4 in]
                      n194 = Equal?(x=w313, y=0) -> (x = y?=w312:bool)
                      n195 = expression code="x*1000000000"(w309) -> (w308:dbl[])
                      n196 = case shown="True" w312 {
                        tunnel: w314 -> [w316 w318]
                        tunnel: [w316 w317] -> w310
                        frame False {
                        }
                        frame True {
                          n197 = Array Size(array=w318) -> (size(s)=w319:i32)
                          n198 = for {
                            N: w319 -> [_]
                            shift-right: [w322] -> _
                            shift-left: w318 -> [w322]
                            tunnel: [w320] -> w317 mode=indexing
                            i -> [w323]
                            n199 = Index Array(array=w322, index=w323) -> (element=w321:dbl)
                            n200 = expression code="10**(x/10)*0.001"(w321) -> (w320:dbl)
                          }
                        }
                      }
                      n201 = local read "Graphs array"() -> (w306:cluster{"ArrayX":dbl[], "ArrayY":dbl[]}[])
                      n202 = Bundle("X array"=w308, "Y array"=w310) -> (w305:cluster{"X array":dbl[], "Y array":dbl[]})  [unwired: 1 in]
                      n203 = Build Array (concatenate)(w306, w305) -> (w304:cluster{"X array":dbl[], "Y array":dbl[]}[])
                      n204 = local write "Graphs array"(w304) -> ()
                      n205 = local write "All spectras"(w304) -> ()
                    }
                    frame #3 {
                      n206 = call <instrlib>:"visa_write+crlf.vi"("error in (no error)"=w324, "Strings (empty)"=":CALCulate" ("write buffer"), "VISA resource name"=w327) -> ("error out"=w325:errorcluster, "VISA resource name out"=w326:refnum<visa-resource-name>)  [unwired: 7 in]
                    }
                    frame #4 {
                      # "smsr"
                      # "2nd peak wl"
                      # "max peak wl"
                      n207 = call <instrlib>:"Read optical power.vi"("error in (no error)"=w357, "VISA resource name"=w358) -> ("error out"=w355:errorcluster, "Optical power"=w347:string, "VISA resource name out"=w356:refnum<visa-resource-name>)  [unwired: 7 in]
                      n208 = local write "VISA out"(w356) -> ()
                      n209 = local write "error out"(w355) -> ()
                      n210 = Spreadsheet String To Array(delimiter (Tab)=",", format string="%.;%f", spreadsheet string=w347, array type (2D Dbl)=dbl[] []) -> (array=w349:dbl[])
                      n211 = Index Array(array=w349, index=0) -> (element=w334:dbl)
                      n212 = Index Array(array=w349, index=2) -> (element=w330:dbl)
                      n213 = Index Array(array=w349, index=5) -> (element=w343:dbl)
                      n214 = Multiply(x=1000000000.0, y=w330) -> (x*y=w329:dbl)
                      n215 = Multiply(x=1000000000.0, y=w334) -> (x*y=w333:dbl)
                      n216 = Build Array (concatenate)(w346, w333) -> (w337:dbl[])
                      n217 = Build Array (concatenate)(w345, w329) -> (w336:dbl[])
                      n218 = Build Array (concatenate)(w344, w343) -> (w335:dbl[])
                      n219 = Bundle("Current meas array"=w339, w337) -> (w342:cluster{"Current meas array":dbl[], dbl[]})  [unwired: 1 in]
                      n220 = Bundle("Current meas array"=w339, w336) -> (w341:cluster{"Current meas array":dbl[], dbl[]})  [unwired: 1 in]
                      n221 = Bundle("Current meas array"=w339, w335) -> (→"SMSR":cluster{"Current meas array":dbl[], dbl[]})  [unwired: 1 in]
                      n222 = Build Array(w342, w341) -> (→"peak wl":cluster{"Current meas array":dbl[], dbl[]}[])
                    }
                    frame #5 {
                      n223 = Divide(x=w364, y=w363) -> (x/y=w361:dbl)
                      n224 = Multiply(x=100.0, y=w361) -> (x*y=w360:dbl)
                      n225 = To Long Integer(number=w360) -> (32bit integer=→"Progress":i32)
                    }
                  }
                }
                n226 = local write "Array 1st peak wl"(w230) -> ()
                n227 = local write "Array smsr"(w231) -> ()
                n228 = local write "Array 2nd peak wl"(w232) -> ()
                n229 = call <instrlib>:"Enable Output.vi"("error in (no error)"=w259, "Enable Output (T: Enable)"=FALSE, "VISA resource name"=w260) -> ("error out"=w254:errorcluster, "VISA resource name out"=w253:refnum<visa-resource-name>)  [unwired: 7 in]
                n230 = call <instrlib>:"Configure Output.vi"("Source Mode  (0: Voltage)"=w257, "error in (no error)"=w254, "Compliance  Level (0.1)"=4.0, "Output Level (0)"=1e-05, "VISA resource name"=w253) -> ("error out"=w236:errorcluster, "VISA resource name out"=w235:refnum<visa-resource-name>)  [unwired: 5 in]
                n231 = VISA Write(VISA resource name=w235, write buffer=":SYST:KEY 23;", error in (no error)=w236) -> (VISA resource name out=w234:refnum<visa-resource-name>, error out=w233:errorcluster)  [unwired: 1 out]
                n232 = call <instrlib>:"Close.vi"("error in (no error)"=w233, "VISA resource name"=w234) -> ("error out"=w237:errorcluster)  [unwired: 9 in]
                n233 = local write "VCSEL error"(w237) -> ()
              }
            }
            n234 = local write "Graphs array"(cluster{"ArrayX":dbl[], "ArrayY":dbl[]}[] [] ("Graphs array")) -> ()
            n235 = local write "Array 1st peak wl"(dbl[] [] ("Array smsr")) -> ()
            n236 = local write "Array 2nd peak wl"(dbl[] [] ("Array smsr")) -> ()
            n237 = local write "Array smsr"(dbl[] [] ("Array smsr")) -> ()
          }
          event "save": Value Change {
            n238 = event-data() -> ()  [unwired: 1 in, 6 out]
            n239 = stacked-sequence {
              frame #0 {
                n240 = case shown="True" "save all spectra data" {
                  frame False {
                  }
                  frame True {
                    n241 = local read "Current meas array"() -> (w376:dbl[])
                    n242 = local read "Graphs array"() -> (w377:cluster{"ArrayX":dbl[], "ArrayY":dbl[]}[])
                    n243 = Number To Fractional String(number=w376, width (-)=i16 20, precision (6)=i16 3) -> (F-format string=w384:string[])  [unwired: 1 in]
                    n244 = for {
                      tunnel: w377 -> [w441] mode=indexing
                      shift-right: [w439] -> w394
                      shift-left: dbl[][] [] -> [w440]
                      tunnel: [w437] -> w373
                      n245 = Unbundle(w441) -> ("ArrayX"=w437:dbl[], "ArrayY"=w438:dbl[])
                      n246 = Build Array (concatenate)(w440, w438) -> (w439:dbl[][])
                    }
                    n247 = for {
                      tunnel: w384 -> [w399] mode=indexing
                      shift-right: [w396] -> w382
                      shift-left: string[] [] -> [w398]
                      n248 = Concatenate Strings(w399, " [mA]" ("string")) -> (w397:string)
                      n249 = Build Array (concatenate)(w398, w397) -> (w396:string[])
                    }
                    n250 = Transpose 2D Array(2D array=w394) -> (transposed array=w385:dbl[][])
                    n251 = Concatenate Strings("Filename all spectra", ".txt" ("string")) -> (w380:string)
                    n252 = Number To Exponential String(number=w385, precision (6)=i16 5, 3:i16 20 ("width (-)")) -> (E-format string=w386:string[][])  [unwired: 1 in]
                    n253 = Build Path(base path="Selecting folder LIV", name or relative path=w380) -> (appended path=w391:path)
                    n254 = Number To Exponential String(number=w373, precision (6)=i16 5, 3:i16 20 ("width (-)")) -> (E-format string=w372:string[])  [unwired: 1 in]
                    n255 = call <vilib>:"Check if File or Folder Exists.vi"("path"=w391) -> ("file or folder exists?"=w392:bool, "dup path"=w381:path)  [unwired: 8 in, 1 out]
                    n256 = Build Array (concatenate)(w382, w386) -> (w370:string[][])
                    n257 = Build Array (concatenate)(" Wavelength, [nm]" ("string"), w372) -> (w366:string[])
                    n258 = Transpose 2D Array(2D array=w370) -> (transposed array=w367:string[][])
                    n259 = Build Array (concatenate)(w366, w367) -> (w369:string[][])
                    n260 = Transpose 2D Array(2D array=w369) -> (transposed array=w368:string[][])
                    "appended array" <- w368
                    n261 = case shown="True" w392 {
                      tunnel: w381 -> [w401 w414]
                      tunnel: w368 -> [w402 w413]
                      frame False {
                        w410 = "" ("Center Button Text (\"No\")")
                        n262 = call-poly <vilib>:"Write To Spreadsheet File.vi"("2D data"=w402, "file path (dialog if empty)"=w401) -> ()  [unwired: 4 in, 3 out]
                        n263 = Path To String(path=w401) -> (string=w403:string)
                        n264 = Concatenate Strings("File successfully saved to" ("string"), "\r", "'" ("Center Button Text (\"No\")"), w403, "'" ("Center Button Text (\"No\")")) -> (w411:string)
                        n265 = call <vilib>:"Three Button Dialog.vi"("Justify Message (Left)"=i16 1 ("precision (6)"), "Window Title (\"\")"="LUI measurement" ("string"), "Right Button Text (\"Cancel\")"=w410, "Center Button Text (\"No\")"=w410, "Left Button Text (\"Yes\")"="Ok" ("Center Button Text (\"No\")"), "message"=w411) -> ()  [unwired: 5 in, 1 out]
                      }
                      frame True {
                        n266 = Path To String(path=w414) -> (string=w421:string)
                        n267 = Concatenate Strings("File '" ("string"), w421, "' already exists." ("string"), "\r", "Do you want to replace file?" ("string")) -> (w424:string)
                        n268 = call <vilib>:"Three Button Dialog.vi"("Justify Message (Left)"=i16 1 ("precision (6)"), "Window Title (\"\")"="LUI measurement" ("string"), "Right Button Text (\"Cancel\")"="" ("Center Button Text (\"No\")"), "message"=w424) -> ("Which Button?"=w415:T2)  [unwired: 7 in]
                        n269 = case shown="\"Left Button\", Default" w415 {
                          tunnel: w414 -> [w434 _]
                          tunnel: w413 -> [w425 _]
                          frame "Left Button", Default {
                            w429 = "" ("Center Button Text (\"No\")")
                            n270 = call-poly <vilib>:"Write To Spreadsheet File.vi"("2D data"=w425, "file path (dialog if empty)"=w434) -> ()  [unwired: 4 in, 3 out]
                            n271 = Path To String(path=w434) -> (string=w433:string)
                            n272 = Concatenate Strings("File successfully replaced as" ("string"), "\r", "'" ("Center Button Text (\"No\")"), w433, "'" ("Center Button Text (\"No\")")) -> (w428:string)
                            n273 = call <vilib>:"Three Button Dialog.vi"("Justify Message (Left)"=i16 1 ("precision (6)"), "Window Title (\"\")"="LUI measurement" ("string"), "Right Button Text (\"Cancel\")"=w429, "Center Button Text (\"No\")"=w429, "Left Button Text (\"Yes\")"="Ok" ("Center Button Text (\"No\")"), "message"=w428) -> ()  [unwired: 5 in, 1 out]
                          }
                          frame "Center Button" {
                          }
                        }
                      }
                    }
                  }
                }
              }
              frame #1 {
                n274 = case shown="True" "save peak wl" {
                  frame False {
                  }
                  frame True {
                    n275 = local read "Current meas array"() -> (w451:dbl[])
                    n276 = local read "Array 2nd peak wl"() -> (w446:dbl[])
                    n277 = local read "Array 1st peak wl"() -> (w450:dbl[])
                    n278 = Number To Fractional String(number=w451, width (-)=i16 20, precision (6)=i16 3) -> (F-format string=w456:string[])  [unwired: 1 in]
                    n279 = Number To Fractional String(number=w450, width (-)=i16 20, precision (6)=i16 3) -> (F-format string=w453:string[])  [unwired: 1 in]
                    n280 = Number To Fractional String(number=w446, width (-)=i16 20, precision (6)=i16 3) -> (F-format string=w447:string[])  [unwired: 1 in]
                    n281 = local read "Selecting folder LIV"() -> (w464:path)
                    n282 = Concatenate Strings("Filename peak wl", ".txt" ("string")) -> (w465:string)
                    n283 = Build Array (concatenate)("Current, mA" ("string"), w456) -> (w457:string[])
                    n284 = Build Array (concatenate)("1st peak, nm" ("element"), w453) -> (w452:string[])
                    n285 = Build Array (concatenate)("2st peak, nm" ("element"), w447) -> (w444:string[])
                    n286 = Build Array(w457, w452, w444) -> (w459:string[][])
                    n287 = Build Path(base path=w464, name or relative path=w465) -> (appended path=w467:path)
                    n288 = Transpose 2D Array(2D array=w459) -> (transposed array=w443:string[][])
                    n289 = call <vilib>:"Check if File or Folder Exists.vi"("path"=w467) -> ("file or folder exists?"=w468:bool, "dup path"=w466:path)  [unwired: 8 in, 1 out]
                    n290 = case shown="True" w468 {
                      tunnel: w466 -> [w470 w483]
                      tunnel: w443 -> [w471 w482]
                      frame False {
                        w479 = "" ("Center Button Text (\"No\")")
                        n291 = call-poly <vilib>:"Write To Spreadsheet File.vi"("2D data"=w471, "file path (dialog if empty)"=w470) -> ()  [unwired: 4 in, 3 out]
                        n292 = Path To String(path=w470) -> (string=w472:string)
                        n293 = Concatenate Strings("File successfully saved to" ("string"), "\r", "'" ("Center Button Text (\"No\")"), w472, "'" ("Center Button Text (\"No\")")) -> (w480:string)
                        n294 = call <vilib>:"Three Button Dialog.vi"("Justify Message (Left)"=i16 1 ("precision (6)"), "Window Title (\"\")"="LUI measurement" ("string"), "Right Button Text (\"Cancel\")"=w479, "Center Button Text (\"No\")"=w479, "Left Button Text (\"Yes\")"="Ok" ("Center Button Text (\"No\")"), "message"=w480) -> ()  [unwired: 5 in, 1 out]
                      }
                      frame True {
                        n295 = Path To String(path=w483) -> (string=w490:string)
                        n296 = Concatenate Strings("File '" ("string"), w490, "' already exists." ("string"), "\r", "Do you want to replace file?" ("string")) -> (w493:string)
                        n297 = call <vilib>:"Three Button Dialog.vi"("Justify Message (Left)"=i16 1 ("precision (6)"), "Window Title (\"\")"="LUI measurement" ("string"), "Right Button Text (\"Cancel\")"="" ("Center Button Text (\"No\")"), "message"=w493) -> ("Which Button?"=w484:T2)  [unwired: 7 in]
                        n298 = case shown="\"Left Button\", Default" w484 {
                          tunnel: w483 -> [w503 _]
                          tunnel: w482 -> [w494 _]
                          frame "Left Button", Default {
                            w498 = "" ("Center Button Text (\"No\")")
                            n299 = call-poly <vilib>:"Write To Spreadsheet File.vi"("2D data"=w494, "file path (dialog if empty)"=w503) -> ()  [unwired: 4 in, 3 out]
                            n300 = Path To String(path=w503) -> (string=w502:string)
                            n301 = Concatenate Strings("File successfully replaced as" ("string"), "\r", "'" ("Center Button Text (\"No\")"), w502, "'" ("Center Button Text (\"No\")")) -> (w497:string)
                            n302 = call <vilib>:"Three Button Dialog.vi"("Justify Message (Left)"=i16 1 ("precision (6)"), "Window Title (\"\")"="LUI measurement" ("string"), "Right Button Text (\"Cancel\")"=w498, "Center Button Text (\"No\")"=w498, "Left Button Text (\"Yes\")"="Ok" ("Center Button Text (\"No\")"), "message"=w497) -> ()  [unwired: 5 in, 1 out]
                          }
                          frame "Center Button" {
                          }
                        }
                      }
                    }
                  }
                }
              }
              frame #2 {
                n303 = case shown="True" "save smsr" {
                  frame False {
                  }
                  frame True {
                    n304 = local read "Current meas array"() -> (w510:dbl[])
                    n305 = local read "Array smsr"() -> (w508:dbl[])
                    n306 = Number To Fractional String(number=w510, width (-)=i16 20, precision (6)=i16 3) -> (F-format string=w515:string[])  [unwired: 1 in]
                    n307 = Number To Fractional String(number=w508, width (-)=i16 20, precision (6)=i16 3) -> (F-format string=w512:string[])  [unwired: 1 in]
                    n308 = local read "Selecting folder LIV"() -> (w522:path)
                    n309 = Concatenate Strings("Filename smsr", ".txt" ("string")) -> (w523:string)
                    n310 = Build Array (concatenate)("Current, mA" ("string"), w515) -> (w516:string[])
                    n311 = Build Array (concatenate)("SMSR, dBm" ("element"), w512) -> (w511:string[])
                    n312 = Build Array(w516, w511) -> (w518:string[][])
                    n313 = Build Path(base path=w522, name or relative path=w523) -> (appended path=w525:path)
                    n314 = Transpose 2D Array(2D array=w518) -> (transposed array=w507:string[][])
                    n315 = call <vilib>:"Check if File or Folder Exists.vi"("path"=w525) -> ("file or folder exists?"=w526:bool, "dup path"=w524:path)  [unwired: 8 in, 1 out]
                    n316 = case shown="True" w526 {
                      tunnel: w524 -> [w528 w541]
                      tunnel: w507 -> [w529 w540]
                      frame False {
                        w537 = "" ("Center Button Text (\"No\")")
                        n317 = call-poly <vilib>:"Write To Spreadsheet File.vi"("2D data"=w529, "file path (dialog if empty)"=w528) -> ()  [unwired: 4 in, 3 out]
                        n318 = Path To String(path=w528) -> (string=w530:string)
                        n319 = Concatenate Strings("File successfully saved to" ("string"), "\r", "'" ("Center Button Text (\"No\")"), w530, "'" ("Center Button Text (\"No\")")) -> (w538:string)
                        n320 = call <vilib>:"Three Button Dialog.vi"("Justify Message (Left)"=i16 1 ("precision (6)"), "Window Title (\"\")"="LUI measurement" ("string"), "Right Button Text (\"Cancel\")"=w537, "Center Button Text (\"No\")"=w537, "Left Button Text (\"Yes\")"="Ok" ("Center Button Text (\"No\")"), "message"=w538) -> ()  [unwired: 5 in, 1 out]
                      }
                      frame True {
                        n321 = Path To String(path=w541) -> (string=w548:string)
                        n322 = Concatenate Strings("File '" ("string"), w548, "' already exists." ("string"), "\r", "Do you want to replace file?" ("string")) -> (w551:string)
                        n323 = call <vilib>:"Three Button Dialog.vi"("Justify Message (Left)"=i16 1 ("precision (6)"), "Window Title (\"\")"="LUI measurement" ("string"), "Right Button Text (\"Cancel\")"="" ("Center Button Text (\"No\")"), "message"=w551) -> ("Which Button?"=w542:T2)  [unwired: 7 in]
                        n324 = case shown="\"Left Button\", Default" w542 {
                          tunnel: w541 -> [w561 _]
                          tunnel: w540 -> [w552 _]
                          frame "Left Button", Default {
                            w556 = "" ("Center Button Text (\"No\")")
                            n325 = call-poly <vilib>:"Write To Spreadsheet File.vi"("2D data"=w552, "file path (dialog if empty)"=w561) -> ()  [unwired: 4 in, 3 out]
                            n326 = Path To String(path=w561) -> (string=w560:string)
                            n327 = Concatenate Strings("File successfully replaced as" ("string"), "\r", "'" ("Center Button Text (\"No\")"), w560, "'" ("Center Button Text (\"No\")")) -> (w555:string)
                            n328 = call <vilib>:"Three Button Dialog.vi"("Justify Message (Left)"=i16 1 ("precision (6)"), "Window Title (\"\")"="LUI measurement" ("string"), "Right Button Text (\"Cancel\")"=w556, "Center Button Text (\"No\")"=w556, "Left Button Text (\"Yes\")"="Ok" ("Center Button Text (\"No\")"), "message"=w555) -> ()  [unwired: 5 in, 1 out]
                          }
                          frame "Center Button" {
                          }
                        }
                      }
                    }
                  }
                }
              }
            }
          }
          event "Exit": Value Change {
            n329 = event-data() -> ()  [unwired: 1 in, 6 out]
            n330 = flat-sequence {
              tunnel: ["Exit"] -> w564
              frame #0 {
                n331 = local read "VISA out"() -> (w567:refnum<visa-resource-name>)
                n332 = local read "error out"() -> (w566:errorcluster)
                n333 = call <instrlib>:"Close.vi"("error in (no error)"=w566, "VISA resource name"=w567) -> ("error out"=w565:errorcluster)  [unwired: 9 in]
                n334 = local write "error out"(w565) -> ()
              }
              frame #1 {
              }
            }
          }
        }
      }
    }
  }
